vi "Revision Query.vi"(0 "VISA Resource Name":refnum<visa-resource-name>, 11 "error in (no error)":errorcluster {"code" format="%.0x"}) -> (4 "VISA Resource Name Out":refnum<visa-resource-name>, 8 "Instr Driver Revision":string, 10 "Instr Firmware Revision":string, 15 "error out":errorcluster {"code" format="%.0x"})   [LabVIEW 2020, in "Olympus IX BX Series.lvlib"]
doc: "This VI queries the current instrument firmware revision and instrument driver revision.\n\nNote: This VI is not supported by the instrument.\n\nThis Instrument Driver's Revision number is 1.1.1.\n\nOlympus Microscope\nCreated By: Karel Pisala\nRelease Date: 8. December 2003\nOriginally Developed in LabVIEW Version: 7.0\n\n\nModification History: \n\nRev 1.0, 12/2003 - Driver Created\n by KP\n\nRev 1.1, 02/2004\nremove:\n OLXXX2 Application Example.vi\nadd application example VIs:\n OLXXX2 Base Example.vi\n OLXXX2 Fluorescence Example BX.vi\n OLXXX2 Objective Example BX.vi\n OLXXX2 Filter Example BX.vi\n OLXXX2 Fluorescence Example IX.vi\n OLXXX2 Objective Example IX.vi\n OLXXX2 Filter Example IX.vi\n\nRev 1.1.1, 09/2004\n Remove bxobjs.mnu menu palette (duplicate and incomplete)"
uses:
  Olympus IX BX Series.lvlib
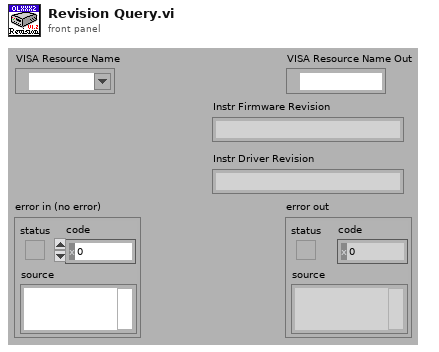
[diagram p1: front panel]
types:
  T1 = cluster{"Status":bool, "Code":i32, "Warning Message:":string}
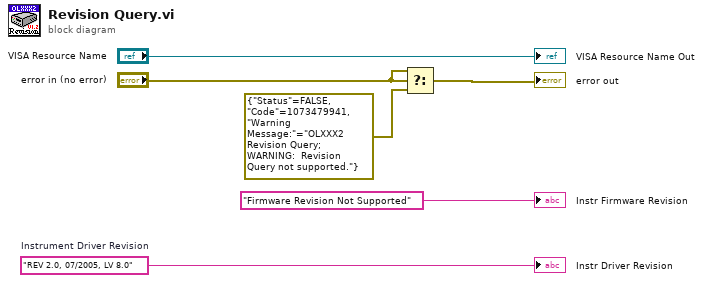
[diagram p0: block diagram]
diagram:
  w6 = "REV 2.0, 07/2005, LV 8.0"  # Instrument Driver Revision
  n1 = Select(t="error in (no error)", s="error in (no error)", f=T1 {"Status"=FALSE, "Code"=1073479941, "Warning Message:"="OLXXX2 Revision Query; WARNING:  Revision Query not supported."}) -> (s? t:f=→"error out":T1)
  "Instr Firmware Revision" <- "Firmware Revision Not Supported"
  "Instr Driver Revision" <- w6
  "VISA Resource Name Out" <- "VISA Resource Name"
